vi "Create Tree Sections from Change List.vi"(8 "error in (no error)":errorcluster, 9 "Database Changes":T1 {"Missing"."Node Ref" format="%.0x"; "Changed"."Old"."Node Ref" format="%.0x"}, 10 "Section":string="Incoming", 11 "TreeControl in":refnum<vi>) -> (0 "error out":errorcluster, 3 "TreeControl out":refnum<vi>)   [LabVIEW 2025, in "Protection and Counter Addon System Explorer.lvlib"]
uses:
  Protection and Counter Addon System Explorer.lvlib
  Types/Database Changes.ctl
  Types/Base Frame Info_NoVS.ctl
  Types/Signal Attributes.ctl
  Types/CAN Filter Type.ctl
  Types/Base Frame Info.ctl
  <vilib>/NI VeriStand/Custom Device API/Custom Device Item Ref.ctl
  Types/Related CAN Frames.ctl
  Types/Related CAN Frames No VS.ctl
  Types/Tree Item Settings.ctl
  <vilib>/Utility/error.llb/Trim Whitespace One-Sided.vi
  <vilib>/NI VeriStand/Custom Device API/Custom Device API.lvlib
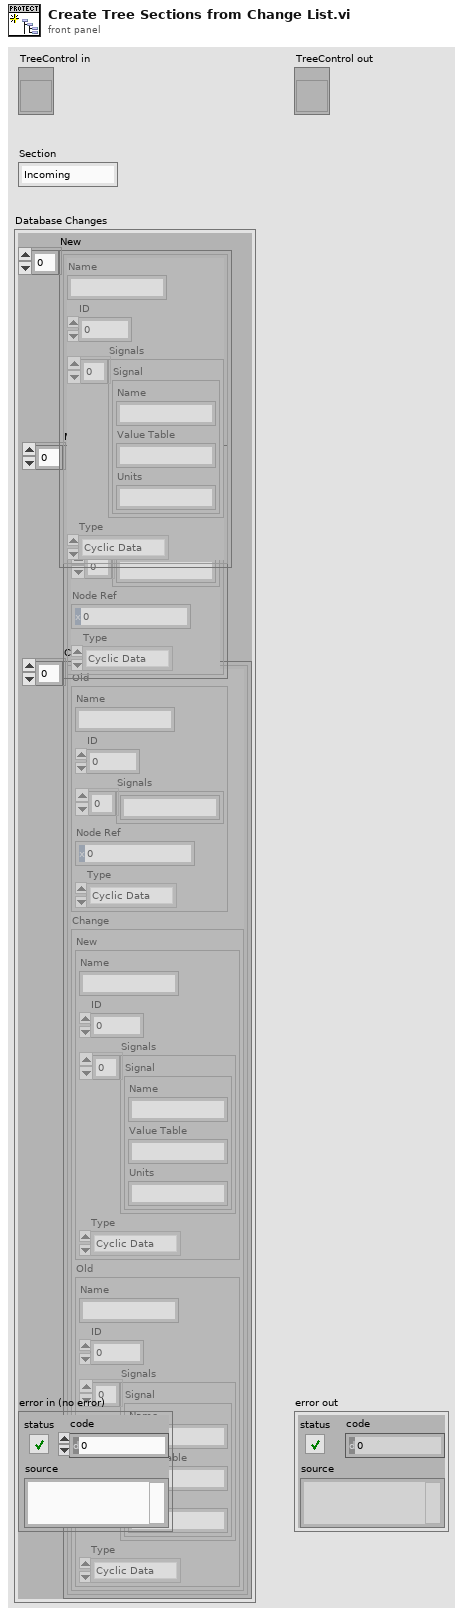
[diagram p1: front panel]
types:
  T1 = typedef "Protection and Counter Addon System Explorer.lvlib/Database Changes.ctl" = cluster{"New":T2[], "Missing":T5[], "Changed":T7[]}
  T2 = typedef "Protection and Counter Addon System Explorer.lvlib/Base Frame Info_NoVS.ctl" = cluster{"Name":string, "ID":u32, "Signals":T3[], "Type":T4}
  T3 = typedef "Protection and Counter Addon System Explorer.lvlib/Signal Attributes.ctl" = cluster{"Name":string, "Value Table":string, "Units":string}
  T4 = typedef "Protection and Counter Addon System Explorer.lvlib/CAN Filter Type.ctl" = enum16{"Cyclic Data", "Event Data", "Cyclic/Event", "All"}
  T5 = typedef "Protection and Counter Addon System Explorer.lvlib/Base Frame Info.ctl" = cluster{"Name":string, "ID":u32, "Signals":string[], "Node Ref":T6, "Type":T4}
  T6 = typedef "Custom Device API.lvlib/Custom Device Item Ref.ctl" = u64
  T7 = typedef "Protection and Counter Addon System Explorer.lvlib/Related CAN Frames.ctl" = cluster{"Old":T5, "Change":T8}
  T8 = typedef "Protection and Counter Addon System Explorer.lvlib/Related CAN Frames No VS.ctl" = cluster{"New":T2, "Old":T2}
  T9 = typedef "Protection and Counter Addon System Explorer.lvlib/Tree Item Settings.ctl" = cluster{"Name":string, "Background Color":u32, "Symbol":i32, "ChildText":string, "Disable":bool}
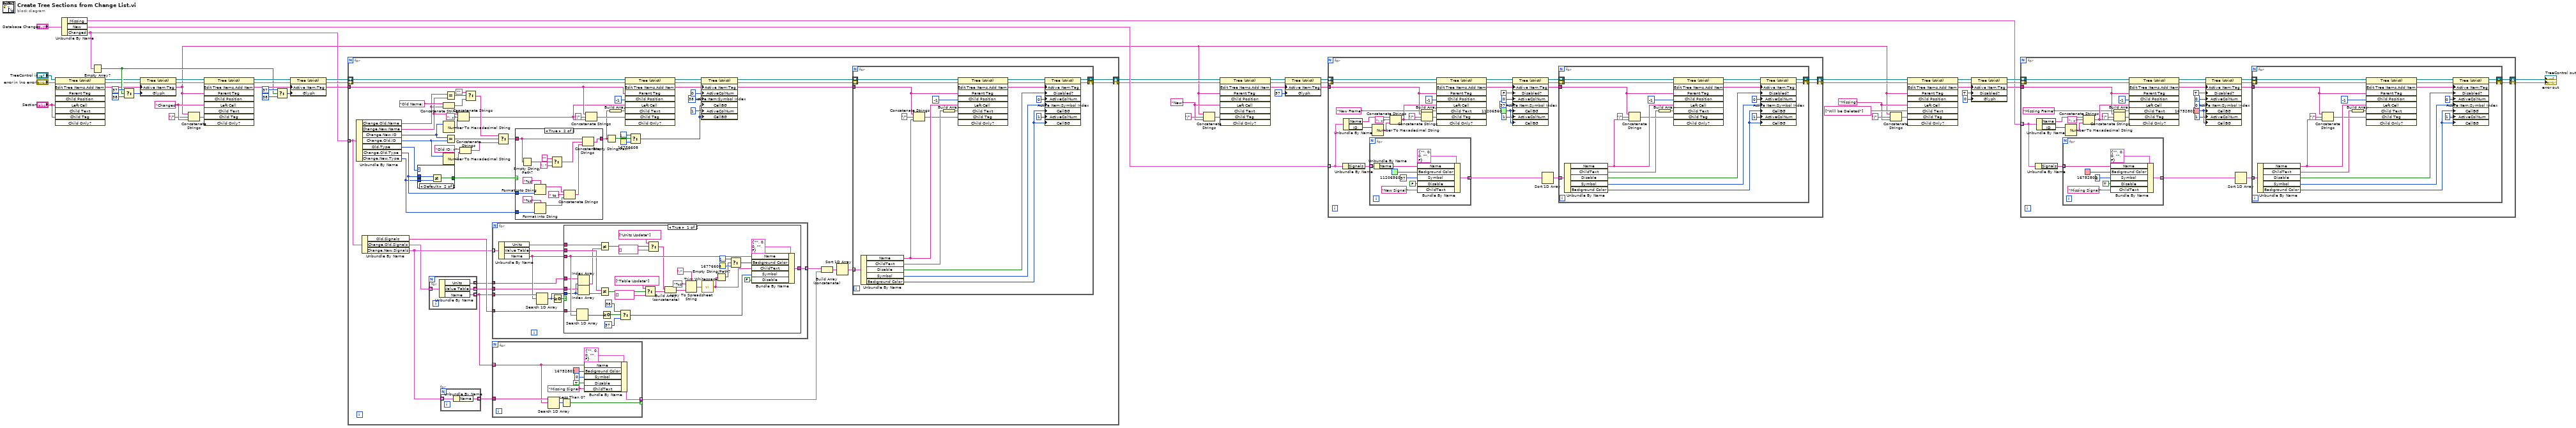
[diagram p0: block diagram]
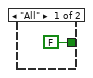
[diagram p2: hidden frame]
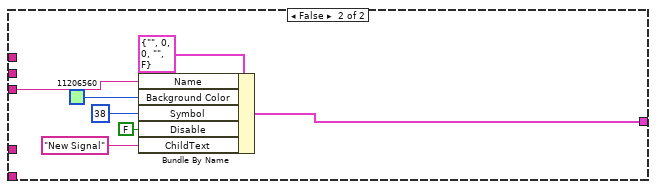
[diagram p4: hidden frame]
diagram:
  w3 = "Missing" ("Parent Tag")
  w6 = "New" ("Parent Tag")
  w22 = "Changed" ("Parent Tag")
  n1 = invoke on="Invoke Node" class="Tree (strict)" method="Edit Tree Items.Add Item"(reference="TreeControl in", error in="error in (no error)", "Left Cell"="Section", "Child Tag"="Section") -> (reference out=w11:refnum<vi>, error out=w9:errorcluster, "Edit Tree Items:Add Item"=w2:string)  [unwired: 5 in, 6 out]
  n2 = Unbundle By Name("Database Changes") -> ("Missing"=w35:T5[], "New"=w30:T2[], "Changed"=w19:T7[])
  n3 = Empty Array?(array=w19) -> (empty?=w12:bool)
  n4 = Select(t=37 ("Active Item:Symbol Index"), s=w12, f=38 ("Active Item:Symbol Index")) -> (s? t:f=w14:i32)
  n5 = property class="Tree (strict)"(reference=w11, error in=w9, "Active Item:Tag"=w2, "Glyph"=w14) -> (reference out=w10:refnum<vi>, error out=w8:errorcluster)
  n6 = Concatenate Strings(w2, "/" ("string"), w22) -> (w20:string)
  n7 = invoke on="Invoke Node" class="Tree (strict)" method="Edit Tree Items.Add Item"(reference=w10, error in=w8, "Parent Tag"=w2, "Left Cell"=w22, "Child Tag"=w20) -> (reference out=w36:refnum<vi>, error out=w37:errorcluster, "Edit Tree Items:Add Item"=w40:string)  [unwired: 4 in, 6 out]
  n8 = Select(t=37 ("Active Item:Symbol Index"), s=w12, f=38 ("Active Item:Symbol Index")) -> (s? t:f=w17:i32)
  n9 = property class="Tree (strict)"(reference=w36, error in=w37, "Active Item:Tag"=w40, "Glyph"=w17) -> (reference out=w39:refnum<vi>, error out=w38:errorcluster)
  n10 = for {
    tunnel: w19 -> [w80] mode=indexing
    shift-right: [w72] -> w28
    shift-left: w38 -> [w89]
    shift-right: [w71] -> w29
    shift-left: w39 -> [w105]
    tunnel: w40 -> [w68]
    n11 = Unbundle By Name(w80) -> ("Change.Old.Name"=w95:string, "Change.New.Name"=w99:string, "Change.New.ID"=w97:u32, "Change.Old.ID"=w101:u32, "Old.Type"=w60:T4, "Change.Old.Type"=w65:T4, "Change.New.Type"=w61:T4)
    n12 = Unbundle By Name(w80) -> ("Old.Signals"=w79:string[], "Change.Old.Signals"=w55:T3[], "Change.New.Signals"=w58:T3[])
    n13 = case shown="Default" w60 {
      tunnel: w65 -> [_ w118]
      tunnel: [FALSE w117] -> w64
      tunnel: w61 -> [_ w116]
      frame "All" {
      }
      frame Default {
        n14 = Not Equal?(x=w118, y=w116) -> (x != y?=w117:bool)
      }
    }
    n15 = for {
      tunnel: w55 -> [w112] mode=indexing
      tunnel: [w111] -> w59 mode=indexing
      tunnel: [w110] -> w56 mode=indexing
      tunnel: [w109] -> w54 mode=indexing
      n16 = Unbundle By Name(w112) -> ("Units"=w109:string, "Value Table"=w110:string, "Name"=w111:string)
    }
    n17 = for {
      tunnel: w58 -> [w114] mode=indexing
      tunnel: [w113] -> w57 mode=indexing
      n18 = Unbundle By Name(w114) -> ("Name"=w113:string)
    }
    n19 = Concatenate Strings("Old Name: ", w95) -> (w90:string)
    n20 = Number To Hexadecimal String(2:w97) -> (0:w96:string)  [unwired: 1 in]
    n21 = Number To Hexadecimal String(2:w101) -> (0:w100:string)  [unwired: 1 in]
    n22 = Equal?(x=w95, y=w99) -> (x = y?=w91:bool)
    n23 = Equal?(x=w97, y=w101) -> (x = y?=w94:bool)
    n24 = Concatenate Strings(w99, ": x" ("string"), w96) -> (w67:string)
    n25 = Concatenate Strings("Old ID: x", w100) -> (w93:string)
    n26 = Select(t="", s=w91, f=w90) -> (s? t:f=w87:string)
    n27 = for {
      tunnel: w59 -> [w174]
      tunnel: w58 -> [w172] mode=indexing
      tunnel: [w173] -> w78 mode=indexing
      tunnel: w79 -> [w169]
      tunnel: w56 -> [w166]
      tunnel: w54 -> [w164]
      n28 = Unbundle By Name(w172) -> ("Units"=w165:string, "Value Table"=w168:string, "Name"=w170:string)
      n29 = Search 1D Array(1D array=w174, element=w170) -> (index of element=w167:i32)  [unwired: 1 in]
      n30 = Greater Or Equal To 0?(x=w167) -> (x >= 0?=w171:bool)
      n31 = case shown="True" w171 {
        tunnel: [w203 w213] -> w173
        tunnel: w170 -> [w199 w209]
        tunnel: w169 -> [w201 _]
        tunnel: w168 -> [w196 _]
        tunnel: w167 -> [w192 _]
        tunnel: w166 -> [w198 _]
        tunnel: w165 -> [w191 _]
        tunnel: w164 -> [w193 _]
        frame True {
          n32 = Search 1D Array(1D array=w201, element=w199) -> (index of element=w202:i32)  [unwired: 1 in]
          n33 = Index Array(array=w193, index=w192) -> (element=w190:string)
          n34 = Index Array(array=w198, index=w192) -> (element=w197:string)
          n35 = Not Equal?(x=w191, y=w190) -> (x != y?=w185:bool)
          n36 = Not Equal?(x=w196, y=w197) -> (x != y?=w194:bool)
          n37 = Greater Or Equal To 0?(x=w202) -> (x >= 0?=w200:bool)
          n38 = Select(t=38 ("Active Item:Symbol Index"), s=w200, f=37 ("Active Item:Symbol Index")) -> (s? t:f=w206:i32)
          n39 = Select(t=string[] ["Table Update"], s=w194, f=string[] []) -> (s? t:f=w183:string[])
          n40 = Select(t=string[] ["Units Update"], s=w185, f=string[] []) -> (s? t:f=w184:string[])
          n41 = Build Array (concatenate)(w184, w183) -> (w182:string[])
          n42 = Array To Spreadsheet String(delimiter (Tab)=";", array=w182, 3:"%s" ("format string")) -> (spreadsheet string=w179:string)
          n43 = call <vilib>:"Trim Whitespace.vi"("string"=w179) -> ("trimmed string"=w175:string)  [unwired: 1 in]
          n44 = Empty String/Path?(string/path=w175) -> (empty?=w176:bool)
          n45 = Select(t=u32 16777216, s=w176, f=u32 16776608) -> (s? t:f=w195:u32)
          n46 = Bundle By Name(cluster=T9 {"Name"="", "Background Color"=0, "Symbol"=0, "ChildText"="", "Disable"=FALSE}, "Name"=w199, "Background Color"=w195, "ChildText"=w175, "Symbol"=w206, "Disable"=FALSE) -> (w203:T9)
        }
        frame False {
          n47 = Bundle By Name(cluster=T9 {"Name"="", "Background Color"=0, "Symbol"=0, "ChildText"="", "Disable"=FALSE}, "Name"=w209, "Background Color"=u32 11206560, "Symbol"=38 ("Active Item:Symbol Index"), "Disable"=FALSE, "ChildText"="New Signal" ("string")) -> (w213:T9)
        }
      }
    }
    n48 = for {
      tunnel: w57 -> [w163]
      tunnel: w59 -> [w154] mode=indexing
      tunnel: [w158] -> w77 mode=indexing if=w161
      n49 = Search 1D Array(1D array=w163, element=w154) -> (index of element=w162:i32)  [unwired: 1 in]
      n50 = Less Than 0?(x=w162) -> (x < 0?=w161:bool)
      n51 = Bundle By Name(cluster=T9 {"Name"="", "Background Color"=0, "Symbol"=0, "ChildText"="", "Disable"=FALSE}, "Name"=w154, "Background Color"=u32 16752802, "Symbol"=0 ("Active Item:Symbol Index"), "Disable"=TRUE, "ChildText"="Missing Signal" ("string")) -> (w158:T9)
    }
    n52 = Select(t=w87, s=w94, f=w93) -> (s? t:f=w63:string)
    n53 = case shown="True" w64 {
      tunnel: w65 -> [_ w133]
      tunnel: [w119 w131] -> w62
      tunnel: w63 -> [w119 w120]
      tunnel: w61 -> [_ w125]
      frame False {
      }
      frame True {
        n54 = Empty String/Path?(string/path=w120) -> (empty?=w130:bool)
        n55 = Format Into String(format string="%s", w133) -> (resulting string=w124:string)  [unwired: 2 in, 1 out]
        n56 = Format Into String(format string="%s", w125) -> (resulting string=w122:string)  [unwired: 2 in, 1 out]
        n57 = Select(t="", s=w130, f="; ") -> (s? t:f=w128:string)
        n58 = Concatenate Strings(w124, " to " ("string"), w122) -> (w121:string)
        n59 = Concatenate Strings(w120, w128, w121) -> (w131:string)
      }
    }
    n60 = Concatenate Strings(w68, "/" ("string"), w67) -> (w66:string)
    n61 = Empty String/Path?(string/path=w62) -> (empty?=w86:bool)
    n62 = Build Array(w62) -> (w88:string[])
    n63 = invoke on="Invoke Node" class="Tree (strict)" method="Edit Tree Items.Add Item"(reference=w105, error in=w89, "Parent Tag"=w68, "Child Position"=-1, "Left Cell"=w67, "Child Text"=w88, "Child Tag"=w66) -> (reference out=w108:refnum<vi>, error out=w107:errorcluster, "Edit Tree Items:Add Item"=w70:string)  [unwired: 2 in, 6 out]
    n64 = Select(t=u32 16777216, s=w86, f=u32 16776608) -> (s? t:f=w81:u32)
    n65 = property class="Tree (strict)"(reference=w108, error in=w107, "Active Item:Tag"=w70, "ActiveColNum"=0 ("Active Cell:Active Column Number"), "Active Item:Symbol Index"=38, "CellBG"=w81, "ActiveColNum"=1 ("Active Cell:Active Column Number"), "CellBG"=w81) -> (reference out=w75:refnum<vi>, error out=w74:errorcluster)
    n66 = Build Array (concatenate)(w78, w77) -> (w76:T9[])
    n67 = Sort 1D Array(array=w76) -> (sorted array=w73:T9[])
    n68 = for {
      shift-right: [w138] -> w71
      shift-left: w75 -> [w151]
      shift-right: [w139] -> w72
      shift-left: w74 -> [w137]
      tunnel: w73 -> [w149] mode=indexing
      tunnel: w70 -> [w150]
      n69 = Unbundle By Name(w149) -> ("Name"=w148:string, "ChildText"=w136:string, "Disable"=w135:bool, "Symbol"=w140:i32, "Background Color"=w134:u32)
      n70 = Concatenate Strings(w150, "/" ("string"), w148) -> (w147:string)
      n71 = Build Array(w136) -> (w146:string[])
      n72 = invoke on="Invoke Node" class="Tree (strict)" method="Edit Tree Items.Add Item"(reference=w151, error in=w137, "Parent Tag"=w150, "Child Position"=-1, "Left Cell"=w148, "Child Text"=w146, "Child Tag"=w147) -> (reference out=w143:refnum<vi>, error out=w142:errorcluster, "Edit Tree Items:Add Item"=w141:string)  [unwired: 2 in, 6 out]
      n73 = property class="Tree (strict)"(reference=w143, error in=w142, "Active Item:Tag"=w141, "Disabled?"=w135, "ActiveColNum"=0 ("Active Cell:Active Column Number"), "Active Item:Symbol Index"=w140, "CellBG"=w134, "ActiveColNum"=1 ("Active Cell:Active Column Number"), "CellBG"=w134) -> (reference out=w138:refnum<vi>, error out=w139:errorcluster)
    }
  }
  n74 = Concatenate Strings(w2, "/" ("string"), w6) -> (w5:string)
  n75 = invoke on="Invoke Node" class="Tree (strict)" method="Edit Tree Items.Add Item"(reference=w29, error in=w28, "Parent Tag"=w2, "Left Cell"=w6, "Child Tag"=w5) -> (reference out=w43:refnum<vi>, error out=w44:errorcluster, "Edit Tree Items:Add Item"=w42:string)  [unwired: 4 in, 6 out]
  n76 = property class="Tree (strict)"(reference=w43, error in=w44, "Active Item:Tag"=w42, "Glyph"=37 ("Active Item:Symbol Index")) -> (reference out=w46:refnum<vi>, error out=w45:errorcluster)
  n77 = for {
    tunnel: w30 -> [w231] mode=indexing
    shift-right: [w226] -> w32
    shift-left: w45 -> [w235]
    shift-right: [w225] -> w31
    shift-left: w46 -> [w241]
    tunnel: w42 -> [w222]
    w218 = u32 11206560
    n78 = Unbundle By Name(w231) -> ("Signals"=w230:T3[])
    n79 = Unbundle By Name(w231) -> ("Name"=w239:string, "ID"=w237:u32)
    n80 = for {
      tunnel: w230 -> [w269] mode=indexing
      tunnel: [w270] -> w217 mode=indexing
      n81 = Unbundle By Name(w269) -> ("Name"=w265:string)
      n82 = Bundle By Name(cluster=T9 {"Name"="", "Background Color"=0, "Symbol"=0, "ChildText"="", "Disable"=FALSE}, "Name"=w265, "Background Color"=u32 11206560, "Symbol"=37 ("Active Item:Symbol Index"), "Disable"=FALSE, "ChildText"="New Signal" ("string")) -> (w270:T9)
    }
    n83 = Number To Hexadecimal String(2:w237) -> (0:w236:string)  [unwired: 1 in]
    n84 = Concatenate Strings(w239, ": x" ("string"), w236) -> (w221:string)
    n85 = Build Array("New Frame" ("string")) -> (w234:string[])
    n86 = Concatenate Strings(w222, "/" ("string"), w221) -> (w220:string)
    n87 = invoke on="Invoke Node" class="Tree (strict)" method="Edit Tree Items.Add Item"(reference=w241, error in=w235, "Parent Tag"=w222, "Child Position"=-1, "Left Cell"=w221, "Child Text"=w234, "Child Tag"=w220) -> (reference out=w244:refnum<vi>, error out=w243:errorcluster, "Edit Tree Items:Add Item"=w224:string)  [unwired: 2 in, 6 out]
    n88 = property class="Tree (strict)"(reference=w244, error in=w243, "Active Item:Tag"=w224, "Disabled?"=FALSE ("Active Item:Disabled?"), "ActiveColNum"=0 ("Active Cell:Active Column Number"), "Active Item:Symbol Index"=37, "CellBG"=w218, "ActiveColNum"=1 ("Active Cell:Active Column Number"), "CellBG"=w218) -> (reference out=w229:refnum<vi>, error out=w228:errorcluster)
    n89 = Sort 1D Array(array=w217) -> (sorted array=w227:T9[])
    n90 = for {
      shift-right: [w249] -> w225
      shift-left: w229 -> [w262]
      shift-right: [w250] -> w226
      shift-left: w228 -> [w248]
      tunnel: w227 -> [w260] mode=indexing
      tunnel: w224 -> [w261]
      n91 = Unbundle By Name(w260) -> ("Name"=w259:string, "ChildText"=w247:string, "Disable"=w246:bool, "Symbol"=w251:i32, "Background Color"=w245:u32)
      n92 = Concatenate Strings(w261, "/" ("string"), w259) -> (w258:string)
      n93 = Build Array(w247) -> (w257:string[])
      n94 = invoke on="Invoke Node" class="Tree (strict)" method="Edit Tree Items.Add Item"(reference=w262, error in=w248, "Parent Tag"=w261, "Child Position"=-1, "Left Cell"=w259, "Child Text"=w257, "Child Tag"=w258) -> (reference out=w254:refnum<vi>, error out=w253:errorcluster, "Edit Tree Items:Add Item"=w252:string)  [unwired: 2 in, 6 out]
      n95 = property class="Tree (strict)"(reference=w254, error in=w253, "Active Item:Tag"=w252, "Disabled?"=w246, "ActiveColNum"=0 ("Active Cell:Active Column Number"), "Active Item:Symbol Index"=w251, "CellBG"=w245, "ActiveColNum"=1 ("Active Cell:Active Column Number"), "CellBG"=w245) -> (reference out=w249:refnum<vi>, error out=w250:errorcluster)
    }
  }
  n96 = Concatenate Strings(w2, "/" ("string"), w3) -> (w1:string)
  n97 = invoke on="Invoke Node" class="Tree (strict)" method="Edit Tree Items.Add Item"(reference=w31, error in=w32, "Parent Tag"=w2, "Left Cell"=w3, "Child Text"=string[] ["Will be Deleted"], "Child Tag"=w1) -> (reference out=w51:refnum<vi>, error out=w49:errorcluster, "Edit Tree Items:Add Item"=w53:string)  [unwired: 3 in, 6 out]
  n98 = property class="Tree (strict)"(reference=w51, error in=w49, "Active Item:Tag"=w53, "Disabled?"=TRUE ("Active Item:Disabled?"), "Glyph"=0 ("Active Item:Symbol Index")) -> (reference out=w52:refnum<vi>, error out=w50:errorcluster)
  n99 = for {
    tunnel: w35 -> [w288] mode=indexing
    shift-right: [w283] -> w34
    shift-left: w50 -> [w292]
    shift-right: [w282] -> w33
    shift-left: w52 -> [w298]
    tunnel: w53 -> [w279]
    w275 = u32 16752802
    n100 = Unbundle By Name(w288) -> ("Signals"=w287:string[])
    n101 = Unbundle By Name(w288) -> ("Name"=w296:string, "ID"=w294:u32)
    n102 = for {
      tunnel: w287 -> [w325] mode=indexing
      tunnel: [w326] -> w274 mode=indexing
      n103 = Bundle By Name(cluster=T9 {"Name"="", "Background Color"=0, "Symbol"=0, "ChildText"="", "Disable"=FALSE}, "Name"=w325, "Background Color"=u32 16752802, "Symbol"=0 ("Active Item:Symbol Index"), "Disable"=TRUE, "ChildText"="Missing Signal" ("string")) -> (w326:T9)
    }
    n104 = Number To Hexadecimal String(2:w294) -> (0:w293:string)  [unwired: 1 in]
    n105 = Concatenate Strings(w296, ": x" ("string"), w293) -> (w278:string)
    n106 = Build Array("Missing Frame" ("string")) -> (w291:string[])
    n107 = Concatenate Strings(w279, "/" ("string"), w278) -> (w277:string)
    n108 = invoke on="Invoke Node" class="Tree (strict)" method="Edit Tree Items.Add Item"(reference=w298, error in=w292, "Parent Tag"=w279, "Child Position"=-1, "Left Cell"=w278, "Child Text"=w291, "Child Tag"=w277) -> (reference out=w301:refnum<vi>, error out=w300:errorcluster, "Edit Tree Items:Add Item"=w281:string)  [unwired: 2 in, 6 out]
    n109 = property class="Tree (strict)"(reference=w301, error in=w300, "Active Item:Tag"=w281, "Disabled?"=TRUE ("Active Item:Disabled?"), "ActiveColNum"=0 ("Active Cell:Active Column Number"), "Active Item:Symbol Index"=0, "CellBG"=w275, "ActiveColNum"=1 ("Active Cell:Active Column Number"), "CellBG"=w275) -> (reference out=w286:refnum<vi>, error out=w285:errorcluster)
    n110 = Sort 1D Array(array=w274) -> (sorted array=w284:T9[])
    n111 = for {
      shift-right: [w306] -> w282
      shift-left: w286 -> [w319]
      shift-right: [w307] -> w283
      shift-left: w285 -> [w305]
      tunnel: w284 -> [w317] mode=indexing
      tunnel: w281 -> [w318]
      n112 = Unbundle By Name(w317) -> ("Name"=w316:string, "ChildText"=w304:string, "Disable"=w303:bool, "Symbol"=w308:i32, "Background Color"=w302:u32)
      n113 = Concatenate Strings(w318, "/" ("string"), w316) -> (w315:string)
      n114 = Build Array(w304) -> (w314:string[])
      n115 = invoke on="Invoke Node" class="Tree (strict)" method="Edit Tree Items.Add Item"(reference=w319, error in=w305, "Parent Tag"=w318, "Child Position"=-1, "Left Cell"=w316, "Child Text"=w314, "Child Tag"=w315) -> (reference out=w311:refnum<vi>, error out=w310:errorcluster, "Edit Tree Items:Add Item"=w309:string)  [unwired: 2 in, 6 out]
      n116 = property class="Tree (strict)"(reference=w311, error in=w310, "Active Item:Tag"=w309, "Disabled?"=w303, "ActiveColNum"=0 ("Active Cell:Active Column Number"), "Active Item:Symbol Index"=w308, "CellBG"=w302, "ActiveColNum"=1 ("Active Cell:Active Column Number"), "CellBG"=w302) -> (reference out=w306:refnum<vi>, error out=w307:errorcluster)
    }
  }
  "error out" <- w34
  "TreeControl out" <- w33
